vi "Write Insert.vi"(8 "error in (no error)":errorcluster, 10 "Abs_Value.lvclass":refnum<class "Abs_Value.lvclass">, 11 "Insert_STR in":refnum<class "Insert_STR.lvclass">) -> (0 "error out":errorcluster, 3 "Insert_STR out":refnum<class "Insert_STR.lvclass">)   [LabVIEW 2021, in "Insert_STR.lvclass"]
uses:
  Insert_STR.lvclass
  Abs_Types/Value/Abs_Value.lvclass
  Insert_STR.lvclass/Insert_STR.ctl
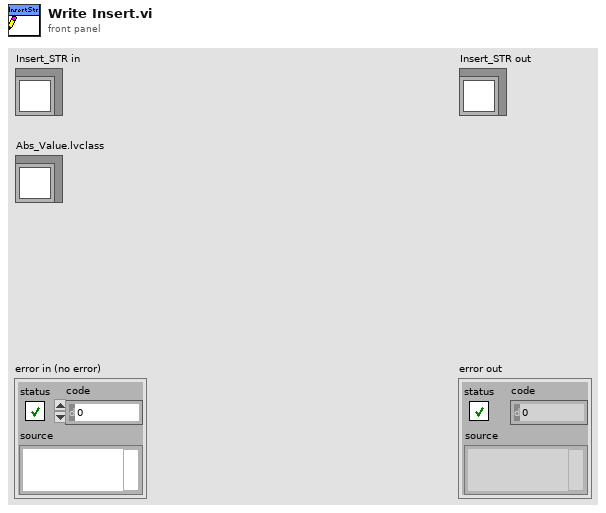
[diagram p1: front panel]
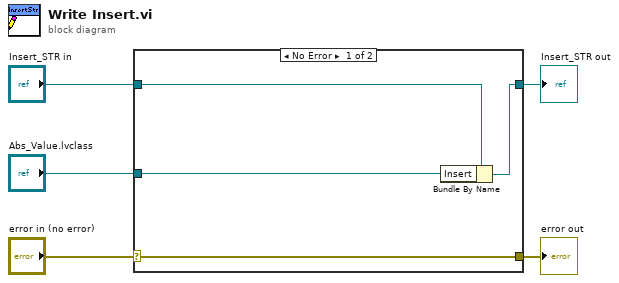
[diagram p0: block diagram]
diagram:
  n1 = case shown="No Error" "error in (no error)" {
    selector: "error in (no error)" -> [w9 w10]
    tunnel: [w9 w10] -> w4
    tunnel: [w7 w11] -> w2
    tunnel: "Insert_STR in" -> [w8 w11]
    tunnel: "Abs_Value.lvclass" -> [w6 _]
    frame No Error {
      n2 = Bundle By Name(cluster=w8, "Insert"=w6) -> (w7:refnum<class "Insert_STR.lvclass">)
    }
    frame Error {
    }
  }
  "error out" <- w4
  "Insert_STR out" <- w2
